vi "RT_encoder_test.vi"() -> ()   [LabVIEW 2017]
uses:
  <vilib>/FPGAPlugInAG/myRIO-1900/niLvFpga_Open_myRIO-1900.vi
  <vilib>/rvi/interface/common/dynamic/niFpgaDynamicAddResources.vi
  <vilib>/Utility/error.llb/Error Cluster From Error Code.vi
  <vilib>/rvi/errors/niLvFpgaAdjustHostInterfaceError.vi
  <vilib>/FPGAPlugInAG/Dynamic/niLvFpga_Close_Dynamic.vi
  <vilib>/rvi/interface/nirviOpenFPGA/nirviOpenFPGA.xnode
  myPAM_FPGATarget_FPGA(TestEncoder_526P0vYbOVg.lvbitx
  FPGA/FPGA (Test Encoders).vi
  <vilib>/rvi/interface/nirviReadWriteControl/nirviReadWriteControl.xnode
  <vilib>/rvi/interface/nirviCloseFPGA/nirviCloseFPGA.xnode
  NiFpgaLv.dll
  <vilib>/rvi/interface/Simulation/niFpgaSimulationCallBeginRW.vi
  <vilib>/ptbypt/NI_PtbyPt.lvlib
panel:
  in  "Forward Coefficients":dbl[](array[numeric])
  in  "Filter type":enum16{"Median", "IFR", "Stavitzky-Golay"}(ring)=enum."Stavitzky-Golay"
  in  "rank":i32=2
  in  "order polynomial":i32=3
  in  "side points":i32=6
  out "speed":cluster{dbl, "Filtered x":dbl}(graph)
  out "Gauge":cluster{dbl, dbl}(knob)={0.0, 22.271095059042633} scale=0.0..360.0
  out "Meter":cluster{dbl, dbl}(knob) scale=0.0..170.0
  in  "stop":bool
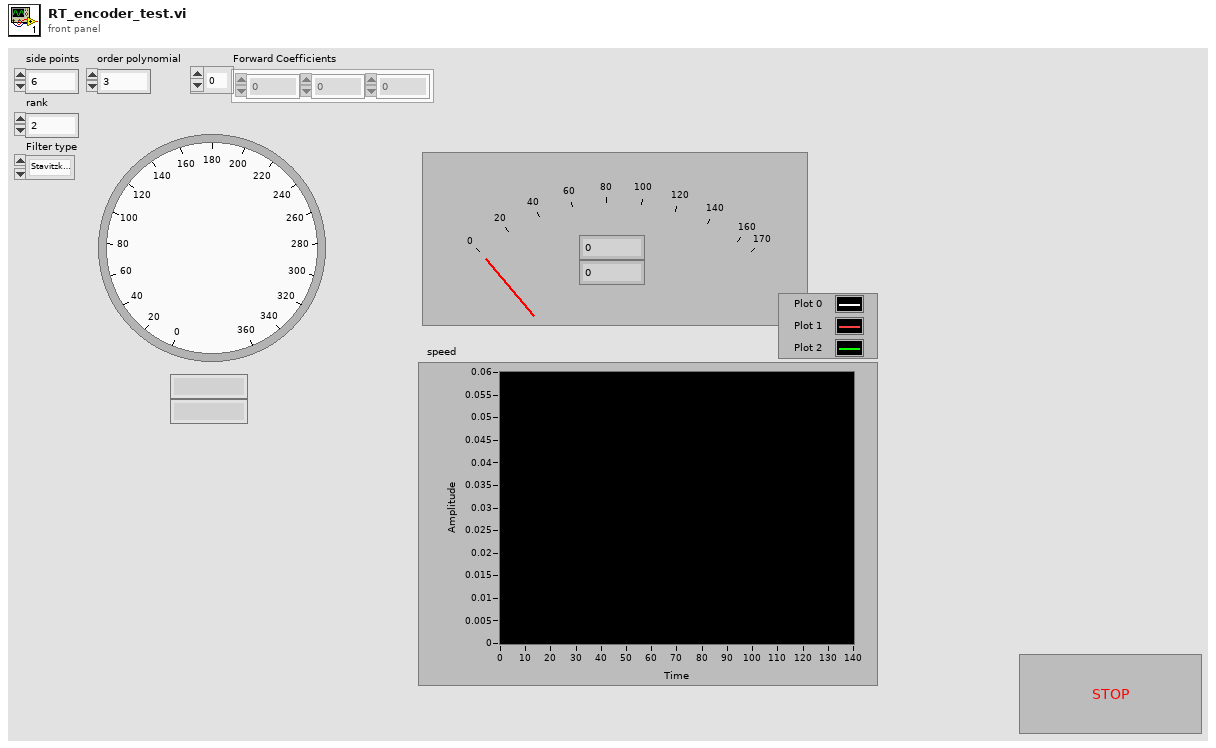
[diagram p1: front panel]
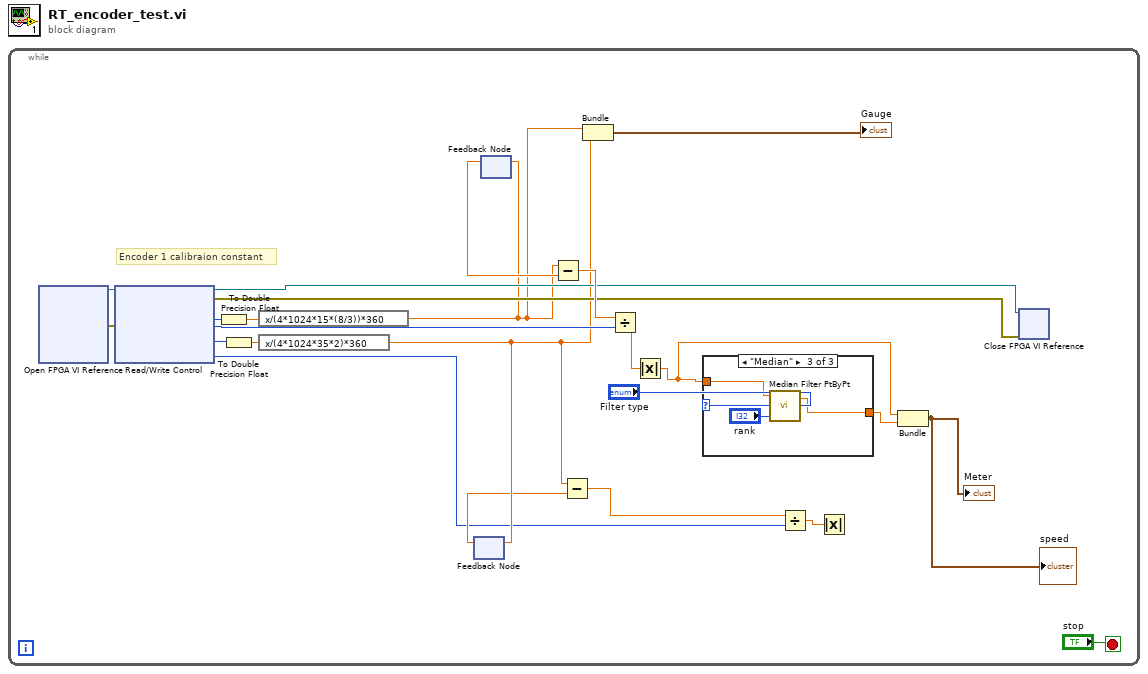
[diagram p0: block diagram]
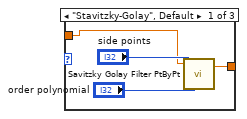
[diagram p2: hidden frame]
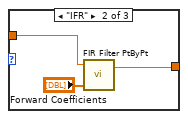
[diagram p3: hidden frame]
diagram:
  n1 = while {
    stop <- "stop" stop-if-true
    # "Encoder 1 calibraion constant"
    n2 = xnode "Open FPGA VI Reference"() -> ("FPGA VI Reference Out"=w23:refnum<k20>, "error out"=w22:errorcluster)  [unwired: 2 in]
    n3 = xnode "Read/Write Control"("FPGA VI Reference In"=w23, "error in"=w22) -> ("FPGA VI Reference Out"=w15:refnum<k20>, "error out"=w14:errorcluster, "Link 1 Counts"=w18:i32, "ENC1_ticks"=w19:i32, "Link 2 Counts 2"=w13:i32, "ENC2_ticks"=w4:i32)
    n4 = To Double Precision Float(number=w18) -> (double precision float=w17:dbl)
    n5 = To Double Precision Float(number=w13) -> (double precision float=w12:dbl)
    n6 = expression code="x/(4*1024*15*(8/3))*360"(w17) -> (w10:dbl)
    n7 = expression code="x/(4*1024*35*2)*360"(w12) -> (w11:dbl)
    n8 = feedback-in #1(w11) -> ()
    n9 = feedback #1() -> (w9:dbl)  [unwired: 1 in]
    n10 = feedback-in #2(w10) -> ()
    n11 = feedback #2() -> (w21:dbl)  [unwired: 1 in]
    n12 = Subtract(x=w10, y=w21) -> (x-y=w20:dbl)
    n13 = Subtract(x=w11, y=w9) -> (x-y=w8:dbl)
    n14 = Bundle(w10, w11) -> (→"Gauge":cluster{dbl, dbl})  [unwired: 1 in]
    n15 = Divide(x=w20, y=w19) -> (x/y=w16:dbl)
    n16 = Absolute Value(x=w16) -> (abs(x)=w1:dbl)
    n17 = case shown="\"Median\"" "Filter type" {
      tunnel: w1 -> [w26 w31 w34]
      tunnel: [w25 w30 w33] -> w2
      frame "Stavitzky-Golay", Default {
        n18 = call <vilib>:"Savitzky Golay Filter PtByPt.vi"("order polynomial"="order polynomial", "side points"="side points", "x"=w26) -> ("Filtered x"=w25:dbl)  [unwired: 1 in, 1 out]
      }
      frame "IFR" {
        n19 = call <vilib>:"FIR Filter PtByPt.vi"("Forward Coefficients"="Forward Coefficients", "x"=w31) -> ("Filtered x"=w30:dbl)  [unwired: 2 in, 1 out]
      }
      frame "Median" {
        n20 = call <vilib>:"Median Filter PtByPt.vi"("rank"="rank", "x"=w34) -> ("Filtered x"=w33:dbl)  [unwired: 2 in, 1 out]
      }
    }
    n21 = Divide(x=w8, y=w4) -> (x/y=w7:dbl)
    n22 = Absolute Value(x=w7) -> ()  [unwired: 1 out]
    n23 = Bundle(w1, "Filtered x"=w2) -> (→"Meter" →"speed":cluster{dbl, "Filtered x":dbl})  [unwired: 1 in]
    n24 = xnode "Close FPGA VI Reference"("FPGA VI Reference In"=w15, "error in"=w14) -> ()  [unwired: 1 out]
  }
